vi "CH_LM FGV Communication Mode.vi"(4 "set? (False)":bool, 5 "error in (no error)":errorcluster, 8 "Communication Mode":T1=enum."USB") -> (0 "error out":errorcluster, 3 "Communication Mode":T1=enum."USB")   [LabVIEW 2017, in "CH_LM.lvlib"]
doc: "This Fuctional Global Variable stores the communication mode in use."
uses:
  CH_LM.lvlib
  CH_LM/CH_LM Communication Mode.ctl
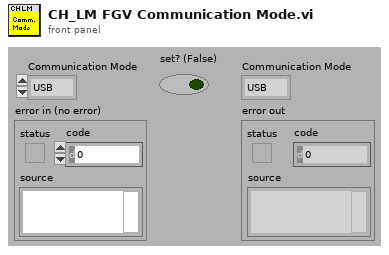
[diagram p1: front panel]
types:
  T1 = typedef "CH_LM.lvlib/CH_LM Communication Mode.ctl" = enum16{"None", "USB", "GPIB", "RS232"}
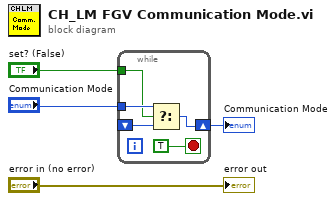
[diagram p0: block diagram]
diagram:
  n1 = while {
    shift-right: [w8] -> w1
    shift-left: _ -> [w9]
    tunnel: "set? (False)" -> [w5]
    tunnel: "Communication Mode" -> [w7]
    stop <- TRUE stop-if-true
    n2 = Select(t=w7, s=w5, f=w9) -> (s? t:f=w8:T1)
  }
  "Communication Mode" <- w1
  "error out" <- "error in (no error)"
